vi "tearDown.vi"(8 "error in (no error)":errorcluster, 11 "reference in":refnum<class "Test mysql.lvclass">) -> (0 "error out":errorcluster, 3 "reference out":refnum<class "Test mysql.lvclass">)   [LabVIEW 2020, in "DataBase_mysql_Tests.lvlib" / "Test mysql.lvclass"]
doc: "tearDown runs after the test method has completed. Use this method to clean up any operations or references that were opened by setUp or the test method. Unit tests should be independent of other unit tests so this VI should ensure that the next test can run in a 'clean' test environment."
uses:
  Test mysql.lvclass
  externals/mysql/Source/mysql.net/mysql.lvclass
  Test mysql.lvclass/Test mysql.ctl
  6a7f7a64-a196-49b6-81da-b722922284b8.vi
  6a7f7a64-a196-49b6-81da-b722922284b8.vi/5136a74e-d4d9-4a1b-b735-d1b214723075.vi
  <vilib>/Utility/error.llb/Error Cluster From Error Code.vi
  externals/database-interface/IDatabase/IDatabase/IDatabase.lvclass
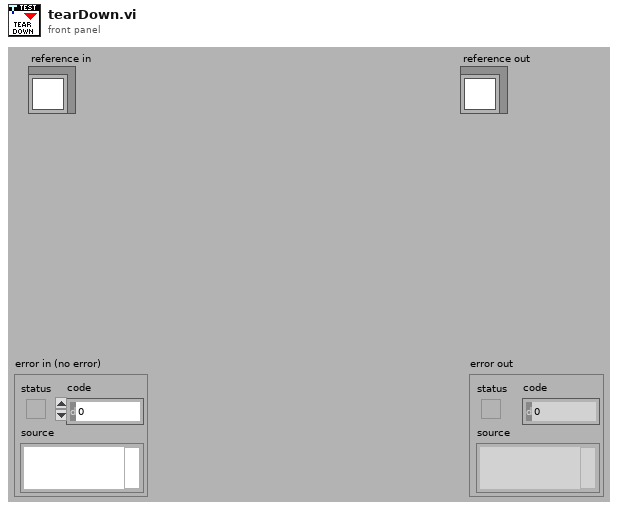
[diagram p1: front panel]
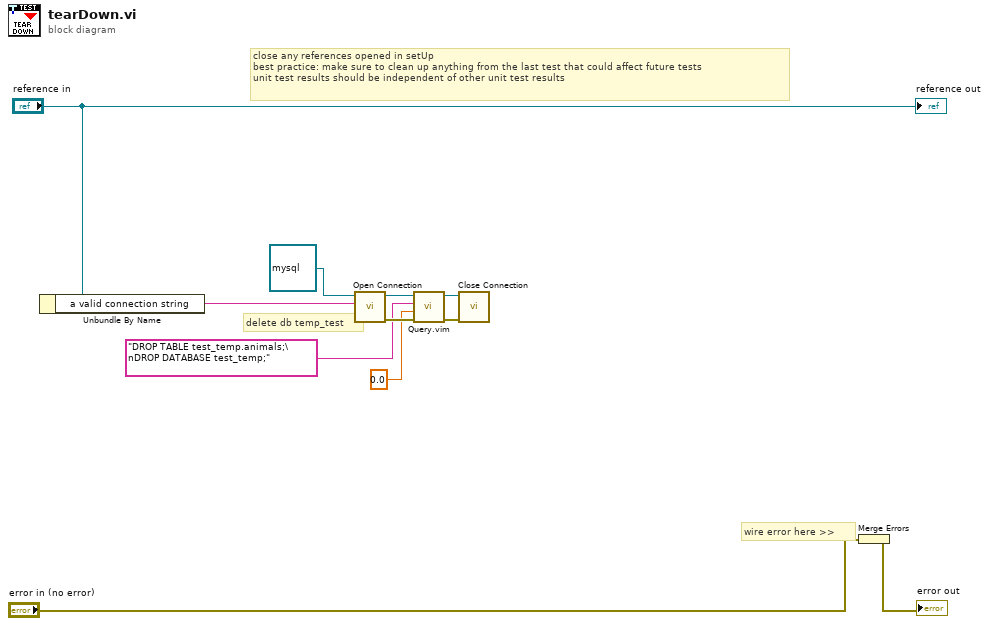
[diagram p0: block diagram]
diagram:
  # "delete db temp_test"
  # "wire error here >>"
  # "close any references opened in setUp\nbest practice: make sure to clean up anything from the last test that could affect future tests\nunit test results should be independent of other unit test results"
  n1 = Unbundle By Name("reference in") -> ("a valid connection string"=w2:string)
  n2 = call-dynamic "Open Connection.vi"("Connection string"=w2, "mysql in"=refnum<class "mysql.lvclass"> refnum) -> ("error out"=w6:errorcluster, "mysql out"=w8:refnum<class "mysql.lvclass">)  [unwired: 8 in]
  n3 = call "Query.vim"("error in (no error)"=w6, "Type and Default"=0.0, "Query string"="DROP TABLE test_temp.animals;\nDROP DATABASE test_temp;", "IDatabase in"=w8) -> ("error out"=w5:errorcluster, "IDatabase out"=w7:refnum<class "mysql.lvclass">)  [unwired: 5 in, 1 out]
  n4 = call-dynamic "Close Connection.vi"("error in (no error)"=w5, "mysql in"=w7) -> ()  [unwired: 8 in, 2 out]
  n5 = Merge Errors("error in (no error)") -> (→"error out":errorcluster)
  "reference out" <- "reference in"
